vi "SDO_TRAJECTORY_EXECUTE_REL.vi"(6 "EnableClosedLoop":bool=TRUE, 8 "Init":bool, 9 "Reverse":bool, 10 "End Relative\nOrientation Deg":dbl, 11 "Gyro Heading\nRAD":dbl) -> (0 "AtReference":bool, 3 "Chassis Velocity Target":T1 {"vOmega" format="%10.3f"; "vY" format="%10.3f"; "vX" format="%10.3f"})   [LabVIEW 2019]
uses:
  <vilib>/Rock Robotics/WPI/ThirdParty/JAS_Junk/TrajLib/TypeDef/CHASSIS_SPEEDS.ctl
  <vilib>/Rock Robotics/WPI/ThirdParty/JAS_Junk/TrajLib/VI/Util_GetTime_U32.vi
  <vilib>/Rock Robotics/WPI/ThirdParty/JAS_Junk/TrajLib/ProfiledPIDController_NewPeriod.vi
  <vilib>/Rock Robotics/WPI/ThirdParty/JAS_Junk/TrajLib/ProfiledPIDController_SetIntegratorRange.vi
  <vilib>/Rock Robotics/WPI/ThirdParty/JAS_Junk/TrajLib/ProfiledPIDController_DisableContInput.vi
  <vilib>/Rock Robotics/WPI/ThirdParty/JAS_Junk/TrajLib/ProfiledPIDController_EnableContInput.vi
  <vilib>/Rock Robotics/WPI/ThirdParty/JAS_Junk/TrajLib/TrapProfConstraint_New.vi
  <vilib>/Rock Robotics/WPI/ThirdParty/JAS_Junk/TrajLib/Conv_Deg_Radians.vi
  <vilib>/Rock Robotics/WPI/ThirdParty/JAS_Junk/TrajLib/Translation2d_Create.vi
  <vilib>/Rock Robotics/WPI/ThirdParty/JAS_Junk/TrajLib/SwerveOdometry_UpdateX.vi
  <vilib>/Rock Robotics/WPI/ThirdParty/JAS_Junk/TrajLib/SwerveOdometry_ResetPosition.vi
  <vilib>/Rock Robotics/WPI/ThirdParty/JAS_Junk/TrajLib/SwerveOdometry_New.vi
  <vilib>/Rock Robotics/WPI/ThirdParty/JAS_Junk/TrajLib/HolDrvCtrl_New.vi
  <vilib>/Rock Robotics/WPI/ThirdParty/JAS_Junk/TrajLib/HolDrvCtrl_PackPID.vi
  <vilib>/Rock Robotics/WPI/ThirdParty/JAS_Junk/TrajLib/HolDrvCtrl_SetTolerance.vi
  <vilib>/Rock Robotics/WPI/ThirdParty/JAS_Junk/TrajLib/HolDrvCtrl_SetEnabled.vi
  <vilib>/Rock Robotics/WPI/ThirdParty/JAS_Junk/TrajLib/HolDrvCtrl_Calculate_Trajectory.vi
  <vilib>/Rock Robotics/WPI/ThirdParty/JAS_Junk/TrajLib/HolDrvCtrl_AtReference.vi
  <vilib>/Rock Robotics/WPI/ThirdParty/JAS_Junk/TrajLib/TrapProfState_New.vi
  <vilib>/Rock Robotics/WPI/ThirdParty/JAS_Junk/TrajLib/PIDController_NewPeriod.vi
  <vilib>/Rock Robotics/SystemInterfaces/NetworkCommunication/NetComm_UsageReport_report.vi
  <vilib>/Rock Robotics/WPI/ThirdParty/JAS_Junk/TrajLib/PIDController_SetIntegratorRange.vi
  <vilib>/Rock Robotics/WPI/ThirdParty/JAS_Junk/TrajLib/PIDController_DisableContinousInput.vi
  <vilib>/Rock Robotics/WPI/ThirdParty/JAS_Junk/TrajLib/PIDController_EnableContinousInput.vi
  <vilib>/Rock Robotics/WPI/ThirdParty/JAS_Junk/TrajLib/Rotation2d_Plus.vi
  <vilib>/Rock Robotics/WPI/ThirdParty/JAS_Junk/TrajLib/Twist2d_Create.vi
  <vilib>/Rock Robotics/WPI/ThirdParty/JAS_Junk/TrajLib/Rotation2d_Minus.vi
  <vilib>/Rock Robotics/WPI/ThirdParty/JAS_Junk/TrajLib/Pose2d_getTranslation.vi
  <vilib>/Rock Robotics/WPI/ThirdParty/JAS_Junk/TrajLib/Pose2d_New_TRRO.vi
  <vilib>/Rock Robotics/WPI/ThirdParty/JAS_Junk/TrajLib/VI/SwerveModulePosition_Get.vi
  <vilib>/Rock Robotics/WPI/ThirdParty/JAS_Junk/TrajLib/VI/SwerveModulePosition_New.vi
  <vilib>/Rock Robotics/WPI/ThirdParty/JAS_Junk/TrajLib/Twist2d_GetAll.vi
  <vilib>/Rock Robotics/WPI/ThirdParty/JAS_Junk/TrajLib/Pose2d_getRotation.vi
  <vilib>/Rock Robotics/WPI/ThirdParty/JAS_Junk/TrajLib/PIDController_Reset.vi
  <vilib>/Rock Robotics/WPI/ThirdParty/JAS_Junk/TrajLib/HolDrvCtrl_Calculate.vi
  <vilib>/Rock Robotics/WPI/ThirdParty/JAS_Junk/TrajLib/Pose2d_getXYAngle.vi
  <vilib>/Rock Robotics/WPI/ThirdParty/JAS_Junk/TrajLib/Rotation2d_GetRadians.vi
  <vilib>/Rock Robotics/WPI/ThirdParty/JAS_Junk/TrajLib/Rotation2d_RotateBy.vi
  <vilib>/Rock Robotics/WPI/ThirdParty/JAS_Junk/TrajLib/Rotation2d_UnaryMinus.vi
  <vilib>/Rock Robotics/WPI/ThirdParty/JAS_Junk/TrajLib/Rotation2d_GetAngleCosSin.vi
  <vilib>/Rock Robotics/WPI/ThirdParty/JAS_Junk/TrajLib/Pose2d_RelativeTo.vi
  <vilib>/Rock Robotics/WPI/ThirdParty/JAS_Junk/TrajLib/ProfiledPIDController_Calculate_Meas_Goal.vi
  <vilib>/Rock Robotics/WPI/ThirdParty/JAS_Junk/TrajLib/ChassisSpeeds_FromFieldRelativeSpeeds.vi
  <vilib>/Rock Robotics/WPI/ThirdParty/JAS_Junk/TrajLib/PIDController_Calculate_SP_PV.vi
  <vilib>/Rock Robotics/WPI/ThirdParty/JAS_Junk/TrajLib/ProfiledPIDController_Reset_PosOnly.vi
  <vilib>/Rock Robotics/WPI/ThirdParty/JAS_Junk/TrajLib/Rotation2d_CreateXY.vi
  <vilib>/Rock Robotics/WPI/ThirdParty/JAS_Junk/TrajLib/Transform2d_Create_PosePose.vi
  <vilib>/Rock Robotics/WPI/ThirdParty/JAS_Junk/TrajLib/ProfiledPIDController_SetGoal_PosOnly.vi
  <vilib>/Rock Robotics/WPI/ThirdParty/JAS_Junk/TrajLib/ProfiledPIDController_Calculate_Meas.vi
  <vilib>/Rock Robotics/WPI/ThirdParty/JAS_Junk/TrajLib/Rotation2d_GetCos.vi
  <vilib>/Rock Robotics/WPI/ThirdParty/JAS_Junk/TrajLib/Rotation2d_GetSin.vi
  <vilib>/Rock Robotics/WPI/ThirdParty/JAS_Junk/TrajLib/PIDController_SetSetpoint.vi
  <vilib>/Rock Robotics/WPI/ThirdParty/JAS_Junk/TrajLib/PIDController_Calculate_PV.vi
  <vilib>/Rock Robotics/WPI/ThirdParty/JAS_Junk/TrajLib/ProfiledPIDController_Reset.vi
  <vilib>/Rock Robotics/WPI/ThirdParty/JAS_Junk/TrajLib/Util_CalcDist.vi
  <vilib>/Rock Robotics/WPI/ThirdParty/JAS_Junk/TrajLib/Translation2d_Minus.vi
  <vilib>/Rock Robotics/WPI/ThirdParty/JAS_Junk/TrajLib/ProfiledPIDController_SetGoal.vi
  <vilib>/Rock Robotics/WPI/ThirdParty/JAS_Junk/TrajLib/TrapProfile_New.vi
  <vilib>/Rock Robotics/WPI/ThirdParty/JAS_Junk/TrajLib/ProfiledPIDController_GetPeriod.vi
  <vilib>/Rock Robotics/WPI/ThirdParty/JAS_Junk/TrajLib/TrapProfile_Calculate.vi
  <vilib>/Rock Robotics/WPI/ThirdParty/JAS_Junk/TrajLib/ControllerUtil_GetModulusError.vi
  <vilib>/Rock Robotics/WPI/ThirdParty/JAS_Junk/TrajLib/TrapProfile_ShouldFlipAcceleration.vi
  <vilib>/Rock Robotics/WPI/ThirdParty/JAS_Junk/TrajLib/TrapProfile_Direct.vi
  <vilib>/Rock Robotics/WPI/ThirdParty/JAS_Junk/TrajLib/PIDController_GetPeriod.vi
  Swerve_Drive_System/SWERVE_DRIVE_GLOBALS.vi
  <vilib>/Rock Robotics/WPI/ThirdParty/JAS_Junk/TrajLib/VI/Util_GetTime_U64.vi
  SDO_TRAJECTORY_GLOBALS.vi
  <vilib>/Rock Robotics/WPI/ThirdParty/JAS_Junk/TrajLib/Globals/Util_LibraryGlobals.vi
  <vilib>/Rock Robotics/WPI/ThirdParty/JAS_Junk/TrajLib/VI/SwerveKinematics_ToTwist2dX.vi
  <vilib>/Rock Robotics/WPI/ThirdParty/JAS_Junk/TrajLib/Pose2d_Exp.vi
  <vilib>/Rock Robotics/WPI/ThirdParty/JAS_Junk/TrajLib/Trajectory_Library.lvlib
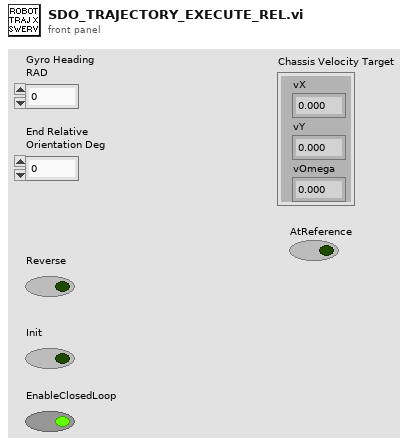
[diagram p1: front panel]
types:
  T1 = typedef "Trajectory_Library.lvlib/CHASSIS_SPEEDS.ctl" = cluster{"vX":dbl, "vY":dbl, "vOmega":dbl}
  T2 = typedef "Trajectory_Library.lvlib/ROTATION2D.ctl" = cluster{"VALUE":dbl, "COS":dbl, "SIN":dbl}
  T3 = typedef "Trajectory_Library.lvlib/SWERVE_DRIVE_KINEMATICS.ctl" = cluster{"NumModules":i32, "InverseKinematics":T4, "ForwardKinematics":T4, "Modules":T5[], "PrevCoR":T5, "SavedModuleStates":T6[]}
  T4 = typedef "NI_Matrix.lvlib/RealMatrix.ctl" = dbl[][]
  T5 = typedef "Trajectory_Library.lvlib/TRANSLATION2D.ctl" = cluster{"X":dbl, "Y":dbl}
  T6 = typedef "Trajectory_Library.lvlib/SWERVE_DRIVE_MODULE_STATE.ctl" = cluster{"Speed":dbl, "Angle":T2}
  T7 = typedef "Trajectory_Library.lvlib/SWERVE_DRIVE_MODULE_POSITION.ctl" = cluster{"Distance":dbl, "Angle":T2, "P":bool}
  T8 = typedef "Trajectory_Library.lvlib/TRAJECTORY.ctl" = cluster{"TotalTImeSecs":dbl, "States":T9[]}
  T9 = typedef "Trajectory_Library.lvlib/TRAJ_STATE.ctl" = cluster{"TimeSeconds":dbl, "Velocity":dbl, "Acceleration":dbl, "POSE":T10, "Curvature":dbl}
  T10 = typedef "Trajectory_Library.lvlib/POSE2D.ctl" = cluster{"TRANSLATION":T5, "ROTATION":T2}
  T11 = typedef "Trajectory_Library.lvlib/PID_TUNING.ctl" = cluster{"Kp":dbl, "Ki":dbl, "Kd":dbl, "MaximumIntegral":dbl, "MinimumIntegral":dbl}
  T12 = typedef "Trajectory_Library.lvlib/PROFILED_PID_CONTROLLER.ctl" = cluster{"Controller":T13, "Goal":T14, "Setpoint":T14, "Constraint":T15}
  T13 = typedef "Trajectory_Library.lvlib/PID_CONTROLLER.ctl" = cluster{"Kp":dbl, "Ki":dbl, "Kd":dbl, "Period":dbl, "Max_Integral":dbl, "Min_Integral":dbl, "Max_Input":dbl, "Min_Input":dbl, "Continuous":bool, "PositionError":dbl, "VelocityError":dbl, "PrevError":dbl, "TotalError":dbl, "PositionTolerance":dbl, "VelocityTolerance":dbl, "SetPoint":dbl, "Kf":dbl, "Prev_Deriv":dbl, "Prev_Deriv 2":dbl, "DerivativeFilter":bool, "Min_Output":dbl, "Max_Output":dbl, "Prev_F_P":dbl, "Prev_F_P_2":dbl, "AntiWindupActive":bool, "Measurement":dbl}
  T14 = typedef "Trajectory_Library.lvlib/TRAPEZOID_PROFILE_STATE.ctl" = cluster{"Position":dbl, "Velocity":dbl}
  T15 = typedef "Trajectory_Library.lvlib/TRAPEZOID_PROFILE_CONSTRAINT.ctl" = cluster{"MaxVelocity":dbl, "MaxAcceleration":dbl}
  T16 = typedef "Trajectory_Library.lvlib/HOLONOMIC_PACK_TUNING.ctl" = cluster{"X PID Tuning":T11, "Y PID Tuning":T11, "thetaProfiledPID_CTRL":T12}
  T17 = typedef "Trajectory_Library.lvlib/HOLONOMIC_DRV_CTRL.ctl" = cluster{"poseTolerance":T10, "poseError":T10, "Enabled":bool, "PID_xCtrl":T13, "PID_yCtrl":T13, "PROF_PID_thetaCtrl":T12, "RotationError":T2, "FirstRun":bool}
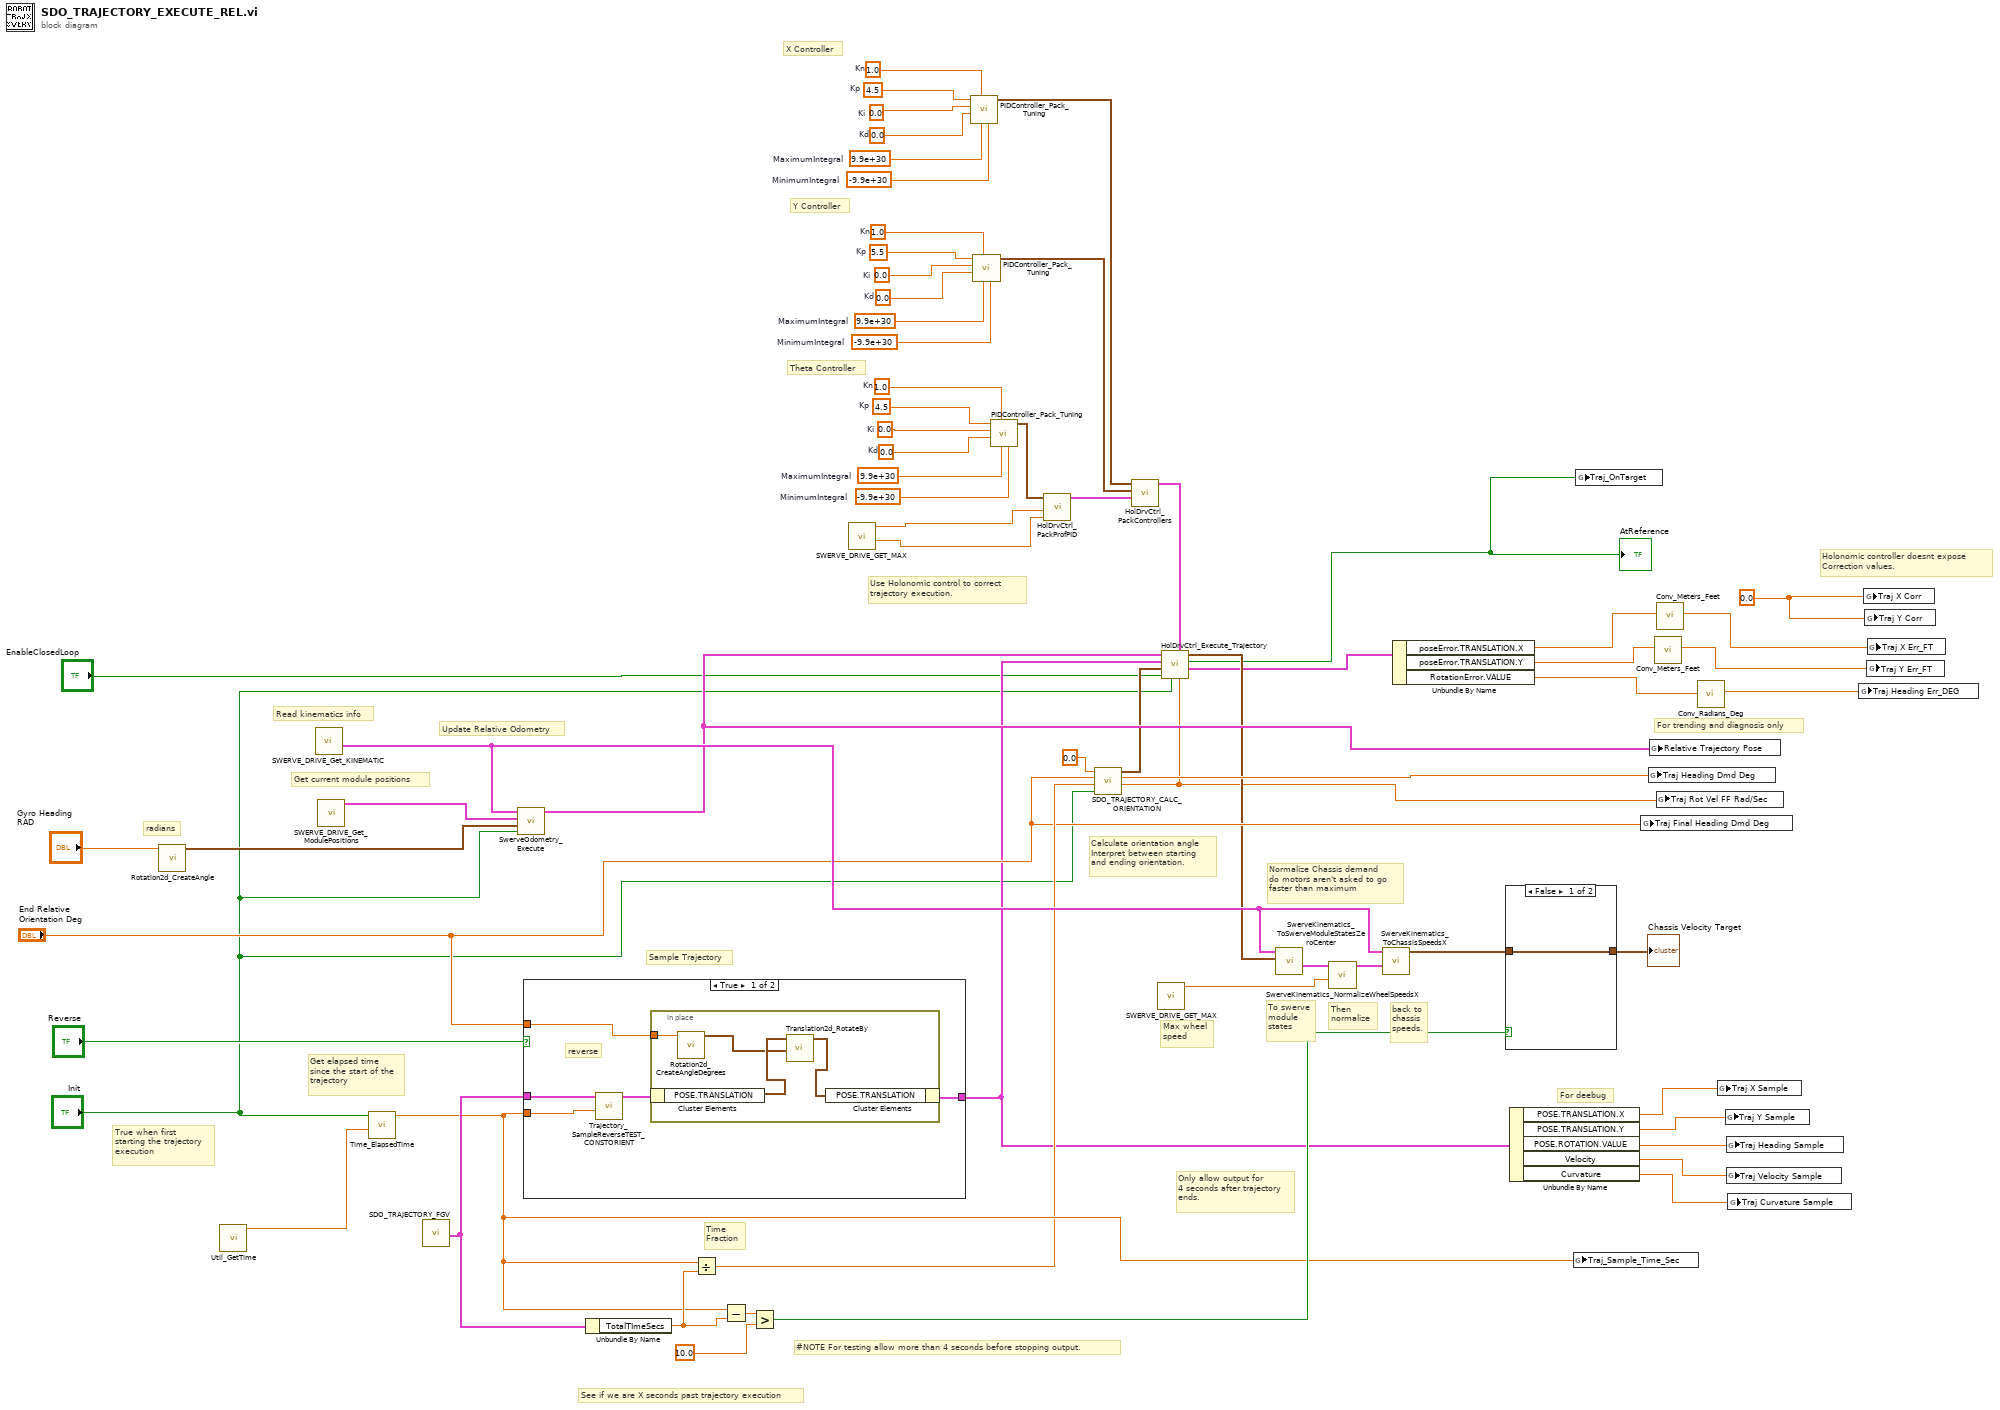
[diagram p0: block diagram]
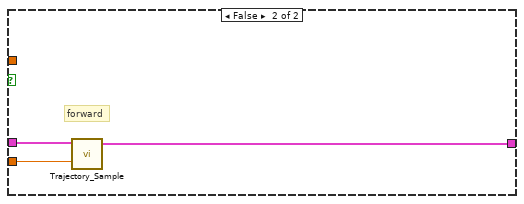
[diagram p2: hidden frame]
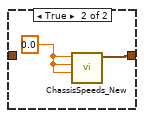
[diagram p3: hidden frame]
diagram:
  w17 = 1.0  # Kn
  w20 = 4.5  # Kp
  w29 = 0.0  # Ki
  w30 = 0.0  # Kd
  w31 = 9.9e+30  # MaximumIntegral
  w32 = -9.9e+30  # MinimumIntegral
  w15 = 1.0  # Kn
  w18 = 4.5  # Kp
  w21 = 0.0  # Ki
  w22 = 0.0  # Kd
  w23 = 9.9e+30  # MaximumIntegral
  w24 = -9.9e+30  # MinimumIntegral
  w16 = 1.0  # Kn
  w19 = 5.5  # Kp
  w25 = 0.0  # Ki
  w26 = 0.0  # Kd
  w27 = 9.9e+30  # MaximumIntegral
  w28 = -9.9e+30  # MinimumIntegral
  w47 = 0.0 ("Y Corr")
  # "Theta Controller"
  # "Y Controller"
  # "X Controller"
  # "Time\nFraction"
  # "Calculate orientation angle\nInterpret between starting\nand ending orientation."
  # "Max wheel\nspeed"
  # "Get current module positions"
  # "True when first\nstarting the trajectory\nexecution"
  # "Get elapsed time\nsince the start of the\ntrajectory"
  # "Holonomic controller doesnt expose\nCorrection values."
  # "Normalize Chassis demand\ndo motors aren't asked to go\nfaster than maximum"
  # "Use Holonomic control to correct\ntrajectory execution."
  # "For trending and diagnosis only"
  # "For deebug"
  # "Update Relative Odometry"
  # "#NOTE For testing allow more than 4 seconds before stopping output."
  # "back to\nchassis\nspeeds."
  # "Then\nnormalize"
  # "To swerve\nmodule\nstates"
  # "Read kinematics info"
  # "Sample Trajectory"
  # "See if we are X seconds past trajectory execution"
  # "radians"
  # "Only allow output for\n4 seconds after trajectory\nends."
  n1 = call <vilib>:"Rotation2d_CreateAngle.vi"("Angle"="Gyro Heading\nRAD") -> ("ROTATION"=w57:T2)  [unwired: 10 in]
  n2 = call <vilib>:"Util_GetTime.vi"() -> ("FPGA_Time_Seconds"=w53:dbl)  [unwired: 9 in, 2 out]
  n3 = call "SWERVE_DRIVE_Get_KINEMATIC.vi"() -> ("out SWERVE_DRIVE_KINEMATICS"=w55:T3)  [unwired: 11 in]
  n4 = call "SWERVE_DRIVE_Get_ModulePositions.vi"() -> ("Swerve Module Positions"=w54:T7[])  [unwired: 11 in]
  n5 = call <vilib>:"Time_ElapsedTime.vi"("PassthroughTime_SEC"=w53, "Reset"="Init") -> ("Elapsed Time Sec"=w44:dbl)  [unwired: 9 in]
  n6 = call "SDO_TRAJECTORY_FGV.vi"() -> ("outTRAJECTORY"=w67:T8)  [unwired: 11 in]
  n7 = call <vilib>:"SwerveOdometry_Execute.vi"("Init"="Init", "Rotation"=w57, "Swerve Module Positions"=w54, "SWERVE_DRIVE_KINEMATICS"=w55) -> ("Current Pose"=w11:T10)  [unwired: 5 in, 2 out]
  n8 = case shown="True" "Reverse" {
    tunnel: w67 -> [w71 w79]
    tunnel: w44 -> [w72 w78]
    tunnel: [w69 w77] -> w10
    tunnel: "End Relative\nOrientation Deg" -> [w68 _]
    frame True {
      # "reverse"
      n9 = call "Trajectory_SampleReverseTEST_CONSTORIENT.vi"("Time"=w72, "InputTRAJECTORY"=w71) -> ("OutputTRAJ_STATE"=w70:T9)  [unwired: 9 in]
      n10 = in-place {
        in-place-border: w68 -> [w74]
        n11 = in-place-cluster #1(w70) -> ("POSE.TRANSLATION"=w75:T5)
        n12 = call <vilib>:"Rotation2d_CreateAngleDegrees.vi"("Angle_Degrees"=w74) -> ("ROTATION"=w73:T2)  [unwired: 10 in]
        n13 = call <vilib>:"Translation2d_RotateBy.vi"("other Rotation"=w73, "In Translation"=w75) -> ("Out Translation"=w76:T5)  [unwired: 9 in]
        n14 = in-place-cluster #1("POSE.TRANSLATION"=w76) -> (w69:T9)
      }
    }
    frame False {
      # "forward"
      n15 = call <vilib>:"Trajectory_Sample.vi"("Time"=w78, "InputTRAJECTORY"=w79) -> ("OutputTRAJ_STATE"=w77:T9)  [unwired: 9 in]
    }
  }
  n16 = Unbundle By Name(w67) -> ("TotalTImeSecs"=w45:dbl)
  n17 = Divide(x=w44, y=w45) -> (x/y=w43:dbl)
  n18 = Subtract(x=w44, y=w45) -> (x-y=w66:dbl)
  n19 = Greater?(x=w66, y=10.0) -> (0:w64:bool)
  n20 = call "SWERVE_DRIVE_GET_MAX.vi"() -> ("Max Rotational Vel (Rad/Sec)"=w12:dbl, "Max Wheel Vel (Meter/Sec)"=w13:dbl)  [unwired: 10 in]
  n21 = call <vilib>:"PIDController_Pack_Tuning.vi"("MinimumIntegral"=w24, "MaximumIntegral"=w23, "Kn"=w15, "Kd"=w22, "Ki"=w21, "Kp"=w18) -> ("PID Tuning"=w33:T11)  [unwired: 5 in]
  n22 = call <vilib>:"PIDController_Pack_Tuning.vi"("MinimumIntegral"=w28, "MaximumIntegral"=w27, "Kn"=w16, "Kd"=w26, "Ki"=w25, "Kp"=w19) -> ("PID Tuning"=w34:T11)  [unwired: 5 in]
  n23 = call <vilib>:"PIDController_Pack_Tuning.vi"("MinimumIntegral"=w32, "MaximumIntegral"=w31, "Kn"=w17, "Kd"=w30, "Ki"=w29, "Kp"=w20) -> ("PID Tuning"=w14:T11)  [unwired: 5 in]
  n24 = call <vilib>:"HolDrvCtrl_PackProfPID.vi"("Max Accel"=w12, "Max Speed"=w13, "Theta PID Tuning"=w14) -> ("Theta PID CONTROLLER"=w35:T12)  [unwired: 8 in]
  n25 = call "SDO_TRAJECTORY_CALC_ORIENTATION.vi"("Init"="Init", "Time Fraction"=w43, "End Orientation Demand DEG"="End Relative\nOrientation Deg", "Starting Orientation  DEG"=0.0) -> ("Rotational Velocity"=w4:dbl, "Orientation Demand Deg"=w46:dbl, "Orientation Demand"=w9:T2)  [unwired: 5 in]
  n26 = call <vilib>:"HolDrvCtrl_PackControllers.vi"("thetaProfiledPID_CTRL"=w35, "Y PID Tuning"=w34, "X PID Tuning"=w33) -> ("HOLONOMIC_CTRL_PACK_TUNING"=w36:T16)  [unwired: 8 in]
  n27 = call "SWERVE_DRIVE_GET_MAX.vi"() -> ("Max Wheel Vel (Meter/Sec)"=w58:dbl)  [unwired: 10 in, 1 out]
  n28 = call <vilib>:"HolDrvCtrl_Execute_Trajectory.vi"("Rotational Velocity Feedforward \nRad/Sec"=w4, "HOLONOMIC_CTRL_PACK_TUNING"=w36, "Reset"="Init", "Enable"="EnableClosedLoop", "angleRef"=w9, "desiredTrajState"=w10, "currentPose"=w11) -> ("outHOLONOMIC_DRV_CTRL"=w6:T17, "AtReference"=w7:bool, "calcChassisSpeed"=w8:T1)  [unwired: 2 in]
  "AtReference" <- w7
  n29 = call <vilib>:"SwerveKinematics_ToSwerveModuleStatesZeroCenter.vi"("ChassisSpeeds"=w8, "in SWERVE_DRIVE_KINEMATICS"=w55) -> ("ModuleStates"=w62:T6[])  [unwired: 8 in, 1 out]
  n30 = call <vilib>:"SwerveKinematics_NormalizeWheelSpeedsX.vi"("AttainableMaxSpeed"=w58, "in WheelStates"=w62) -> ("out WheelStates"=w61:T6[])  [unwired: 9 in]
  n31 = call <vilib>:"SwerveKinematics_ToChassisSpeedsX.vi"("WheelStates"=w61, "in SWERVE_DRIVE_KINEMATICS"=w55) -> ("Chassis Speed"=w56:T1)  [unwired: 9 in]
  n32 = Unbundle By Name(w6) -> ("poseError.TRANSLATION.X"=w40:dbl, "poseError.TRANSLATION.Y"=w39:dbl, "RotationError.VALUE"=w2:dbl)
  n33 = case shown="False" w64 {
    tunnel: w56 -> [w80 _]
    tunnel: [w80 w81] -> w59
    frame False {
    }
    frame True {
      w82 = 0.0 ("vX")
      n34 = call <vilib>:"ChassisSpeeds_New.vi"("vAngular"=w82, "vY"=w82, "vX"=w82) -> ("CHASSIS"=w81:T1)  [unwired: 8 in]
    }
  }
  "Chassis Velocity Target" <- w59
  n35 = Unbundle By Name(w10) -> ("POSE.TRANSLATION.X"=w52:dbl, "POSE.TRANSLATION.Y"=w51:dbl, "POSE.ROTATION.VALUE"=w50:dbl, "Velocity"=w49:dbl, "Curvature"=w48:dbl)
  n36 = global write "SDO_TRAJECTORY_GLOBALS.vi" "Traj_Sample_Time_Sec"(w44) -> ()
  n37 = global write "SDO_TRAJECTORY_GLOBALS.vi" "Traj_OnTarget"(w7) -> ()
  n38 = global write "SDO_TRAJECTORY_GLOBALS.vi" "Traj Final Heading Dmd Deg"("End Relative\nOrientation Deg") -> ()
  n39 = global write "SDO_TRAJECTORY_GLOBALS.vi" "Traj Heading Dmd Deg"(w46) -> ()
  n40 = global write "SDO_TRAJECTORY_GLOBALS.vi" "Relative Trajectory Pose"(w11) -> ()
  n41 = call <vilib>:"Conv_Meters_Feet.vi"("Meters"=w39) -> ("Feet"=w38:dbl)  [unwired: 10 in]
  n42 = call <vilib>:"Conv_Meters_Feet.vi"("Meters"=w40) -> ("Feet"=w37:dbl)  [unwired: 10 in]
  n43 = global write "SDO_TRAJECTORY_GLOBALS.vi" "Traj Rot Vel FF Rad/Sec"(w4) -> ()
  n44 = call <vilib>:"Conv_Radians_Deg.vi"("Radians"=w2) -> ("Degrees"=w41:dbl)  [unwired: 10 in]
  n45 = global write "SDO_TRAJECTORY_GLOBALS.vi" "Traj X Sample"(w52) -> ()
  n46 = global write "SDO_TRAJECTORY_GLOBALS.vi" "Traj Y Sample"(w51) -> ()
  n47 = global write "SDO_TRAJECTORY_GLOBALS.vi" "Traj Heading Sample"(w50) -> ()
  n48 = global write "SDO_TRAJECTORY_GLOBALS.vi" "Traj Velocity Sample"(w49) -> ()
  n49 = global write "SDO_TRAJECTORY_GLOBALS.vi" "Traj Curvature Sample"(w48) -> ()
  n50 = global write "SDO_TRAJECTORY_GLOBALS.vi" "Traj Heading Err_DEG"(w41) -> ()
  n51 = global write "SDO_TRAJECTORY_GLOBALS.vi" "Traj X Corr"(w47) -> ()
  n52 = global write "SDO_TRAJECTORY_GLOBALS.vi" "Traj Y Corr"(w47) -> ()
  n53 = global write "SDO_TRAJECTORY_GLOBALS.vi" "Traj Y Err_FT"(w38) -> ()
  n54 = global write "SDO_TRAJECTORY_GLOBALS.vi" "Traj X Err_FT"(w37) -> ()
